vi "On Mouse Move.vi"(8 "error in (no error)":errorcluster, 10 "Coords":T1, 11 "Interaction in":refnum<class "Interaction.lvclass">) -> (0 "error out":errorcluster, 3 "Interaction out":refnum<class "Interaction.lvclass">)   [LabVIEW 2021, in "Interaction.lvclass"]
doc: "Copyright 2018, Wiebe Walstra, wiebe@carya.nl."
uses:
  Interaction.lvclass
  <vilib>/Utility/miscctls.llb/LVPoint32TypeDef.ctl
  Interaction.lvclass/Interaction.ctl
  Interaction Splitter.lvclass
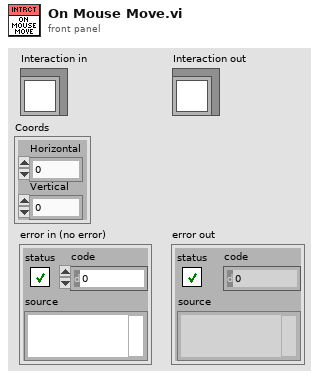
[diagram p1: front panel]
types:
  T1 = typedef "LVPoint32TypeDef.ctl" = cluster{"Horizontal":i32, "Vertical":i32}
  T2 = cluster{"Left":dbl, "Top":dbl, "Right":dbl, "Bottom":dbl}
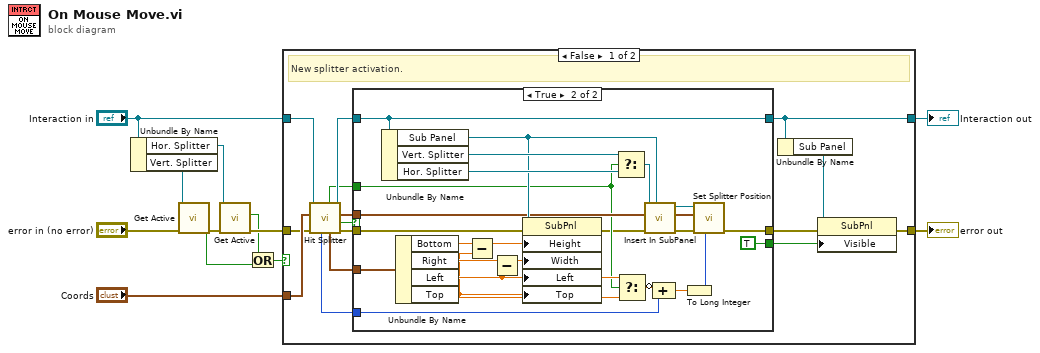
[diagram p0: block diagram]
diagram:
  n1 = Unbundle By Name("Interaction in") -> ("Hor. Splitter"=w4:refnum<class "Interaction Splitter.lvclass">, "Vert. Splitter"=w8:refnum<class "Interaction Splitter.lvclass">)
  n2 = call "Get Active.vi"("error in (no error)"="error in (no error)", "Interaction Splitter in"=w8) -> ("error out"=w7:errorcluster, "Active?"=w3:bool)  [unwired: 7 in, 1 out]
  n3 = call "Get Active.vi"("error in (no error)"=w7, "Interaction Splitter in"=w4) -> ("error out"=w9:errorcluster, "Active?"=w2:bool)  [unwired: 7 in, 1 out]
  n4 = Or(x=w2, y=w3) -> (x .or. y?=w1:bool)
  n5 = case shown="False" w1 {
    tunnel: "Coords" -> [w27 _]
    tunnel: [w15 w55] -> w11
    tunnel: [w18 w54] -> w10
    tunnel: "Interaction in" -> [w23 w55]
    tunnel: w9 -> [w26 w54]
    frame False {
      # "New splitter activation."
      n6 = call-dynamic "Hit Splitter.vi"("error in (no error)"=w26, "Point32"=w27, "IContainer in"=w23) -> ("error out"=w25:errorcluster, "Hit?"=w21:bool, "Limits"=w14:cluster{"Left":i16, "Right":i16}, "IContainer out"=w24:refnum<class "Interaction.lvclass">, "Slider"=w19:T2, "vertical?"=w22:bool, "Position"=w20:i16)  [unwired: 2 in]
      n7 = case shown="True" w21 {
        tunnel: w25 -> [w29 w44]
        tunnel: w24 -> [w28 w45]
        tunnel: [w28 w45] -> w15
        tunnel: w22 -> [_ w36]
        tunnel: [w29 w33] -> w13
        tunnel: w20 -> [_ w42]
        tunnel: w19 -> [_ w46]
        tunnel: [_ TRUE] -> w16
        tunnel: w14 -> [_ w37]
        frame False {
        }
        frame True {
          n8 = Unbundle By Name(w45) -> ("Sub Panel"=w47:refnum<vi>, "Vert. Splitter"=w49:refnum<class "Interaction Splitter.lvclass">, "Hor. Splitter"=w48:refnum<class "Interaction Splitter.lvclass">)
          n9 = Unbundle By Name(w46) -> ("Bottom"=w53:dbl, "Right"=w51:dbl, "Left"=w43:dbl, "Top"=w35:dbl)
          n10 = Subtract(x=w53, y=w35) -> (x-y=w52:dbl)
          n11 = Subtract(x=w51, y=w43) -> (x-y=w50:dbl)
          n12 = property class="SubPnl"(reference=w47, error in=w44, "Height"=w52, "Width"=w50, "Left"=w43, "Top"=w35) -> (error out=w34:errorcluster)  [unwired: 1 out]
          n13 = Select(t=w49, s=w36, f=w48) -> (s? t:f=w31:refnum<class "Interaction Splitter.lvclass">)
          n14 = Select(t=w43, s=w36, f=w35) -> (s? t:f=w41:dbl)
          n15 = call "Insert In SubPanel.vi"("SubPanel"=w47, "error in (no error)"=w34, "Interaction Splitter in"=w31) -> ("error out"=w32:errorcluster, "Interaction Splitter out"=w30:refnum<class "Interaction Splitter.lvclass">)  [unwired: 7 in]
          n16 = Compound Arithmetic op=ADD(invert w41, w42) -> (w40:dbl)
          n17 = To Long Integer(number=w40) -> (32bit integer=w38:i32)
          n18 = call "Set Splitter Position.vi"("Splitter Position"=w38, "error in (no error)"=w32, "Limits"=w37, "Interaction Splitter in"=w30) -> ("error out"=w33:errorcluster)  [unwired: 6 in, 1 out]
        }
      }
      n19 = Unbundle By Name(w15) -> ("Sub Panel"=w17:refnum<vi>)
      n20 = property class="SubPnl"(reference=w17, error in=w13, "Visible"=w16) -> (error out=w18:errorcluster)  [unwired: 1 out]
    }
    frame True {
      # "Splitter is being dragged!"
    }
  }
  "error out" <- w10
  "Interaction out" <- w11
